vi "SetArmControlState.vi"(2 "ArmControlState":string) -> ()   [LabVIEW 2017]
uses:
  <vilib>/Rock Robotics/Network Tables/NT Write String.vi
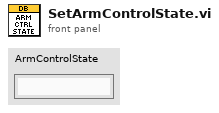
[diagram p1: front panel]
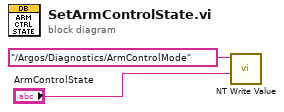
[diagram p0: block diagram]
diagram:
  n1 = call-poly <vilib>:"NT Write Value.vi"("String"="ArmControlState", "Name"="/Argos/Diagnostics/ArmControlMode") -> ()  [unwired: 9 in, 1 out]
